vi "SV UFF58 Format ASCII Function (Complex Spectrum) (1 Ch).vi"(1 "ID lines (1-3)":T9, 2 "data precision (DBL:1)":T11=1 items=["single-precision", "double-precision"], 5 "real part":T10, 7 "imaginary part":T10, 9 "spectrum info":T1={"channel name"="", "description"="", "x-axis units"=0, "spectral info"={"spectrum type"=enum."Power [Magnitude^2]", "linear/dB"=enum."linear", "window"=0, "window size"=0, "FFT size"=0}, "engineering units"=0, "custom label"="", "dB reference [EU]"=0.0, "peak units"=enum."rms", "weighting filter"=0, "spectral density?"=FALSE, "unit label"="", "spectrum skewed?"=FALSE, "complimentary spectrum units"=enum."none"} {"x-axis units" items=["Time (s)"=0, "Frequency-CB (Hz)"=1, "Frequency-CPB (Hz)"=1248, "Frequency-Arbitrary (Hz)"=2357, "Quefrency (s)"=2, "Revolutions (rev)"=3, "Order"=4, "Speed (RPM)"=11, "Speed (rad/s)"=21, "Index"=65535]; "weighting filter" items=["Linear", "A-weighting", "B-weighting", "C-weighting", "ITU-R 468-4", "Dolby", "CCITT", "C-message", "Wb", "Wc", "Wd", "We", "Wf", "Wh", "Wj", "Wk", "Wm", "AES17 20 kHz lowpass", "AES17 40 kHz lowpass", "AES17 20 kHz highpass", "AES17 40 kHz highpass"]; "dB reference [EU]" format="%.2f"; "engineering units" items=["custom..."=0, "V"=1, "A"=21, "C"=30, "pC"=31, "s"=32, "-"=29, "Pa"=2, "N"=20, "g"=3, "m/s^2"=4, "m/s"=5, "m"=6, "mm/s"=12, "mm"=13, "micron/s"=14, "micron"=15, "in/s^2"=7, "in/s"=8, "in"=9, "mil/s"=10, "mil"=11, "rad/s^2"=16, "rad/s"=17, "rad"=18, "deg/s^2"=26, "deg/s"=27, "deg"=28, "RPM"=22, "cycle/s^2"=23, "Hz"=24, "cycle"=25, "strain"=19]; "spectral info"."window" items=["None "=0, "Hanning"=1, "Hamming"=2, "Blackman-Harris"=3, "Exact Blackman"=4, "Blackman"=5, "Flat Top"=6, "4 Term B-Harris "=7, "7 Term B-Harris"=8, "Low Sidelobe"=9, "Force - Exponential"=10, "Gaussian"=62]}, 11 "error in (no error)":errorcluster, 12 "DOF Identification":T8 {"reference direction" items=["-Z Rotation"=-6, "-Y Rotation"=-5, "-X Rotation"=-4, "-Z Translation"=-3, "-Y Translation"=-2, "-X Translation"=-1, "Scalar"=0, "+X Translation"=1, "+Y Translation"=2, "+Z Translation"=3, "+X Rotation"=4, "+Y Rotation"=5, "+Z Rotation"=6]; "response direction" items=["-Z Rotation"=-6, "-Y Rotation"=-5, "-X Rotation"=-4, "-Z Translation"=-3, "-Y Translation"=-2, "-X Translation"=-1, "Scalar"=0, "+X Translation"=1, "+Y Translation"=2, "+Z Translation"=3, "+X Rotation"=4, "+Y Rotation"=5, "+Z Rotation"=6]}) -> (6 "UFF58 ASCII function string":string, 15 "error out":errorcluster)   [LabVIEW 2017, in "SoundVib_UFF58.lvlib"]
doc: "Formats data to the UFF58 (universal file format) ASCII format. This VI also writes the fields in records 1, 2, and 3, <B>ID lines (1-3)</B> as well as all the records and fields associated with the specified instance and the attributes of input data. You can write a single time domain waveform, a single real frequency spectrum, or a complex frequency spectrum to a UFF58 formatted string. If a frequency spectrum is in decibels, this VI converts the spectrum to linear before writing the data to the formatted string. The default instance, SV UFF58 Format ASCII Function (Time Waveform), writes a single time domain waveform to the file specified by the <B>waveform</B> input. Wire data to the <B>waveform</B> input to determine the polymorphic instance to use or manually select the instance."
uses:
  <vilib>/addons/Sound and Vibration/svt_UFF58/SoundVib_UFF58.lvlib
  <vilib>/addons/Sound and Vibration/svt_UFF58/subVIs/sv_UFF58 Data Precision.ctl
  <vilib>/addons/Sound and Vibration/svt_UFF58/subVIs/sv_IDLines123.ctl
  <vilib>/addons/Sound and Vibration/svt_UFF58/subVIs/sv_UFF58 Response Direction.ctl
  <vilib>/addons/_NISVFA/_Shared subVIs/Controls/svc_Spectrum Info.ctl
  <vilib>/addons/_NISVFA/_Shared subVIs/Controls/svc_X-Axis Units.ctl
  <vilib>/addons/_NISVFA/_Shared subVIs/Controls/svc_Spectrum Type.ctl
  <vilib>/addons/_NISVFA/_Shared subVIs/Controls/svc_Engineering Units Text Ring.ctl
  <vilib>/addons/_NISVFA/_Shared subVIs/Controls/svc_Weighting Filter Text Ring.ctl
  <vilib>/addons/_NISVFA/_Shared subVIs/Controls/svc_Complimentary Spectrum Units.ctl
  <vilib>/addons/Sound and Vibration/svt_UFF58/subVIs/sv_UFF58 Check Data Valid (Freq - Complex) (1 Ch).vi
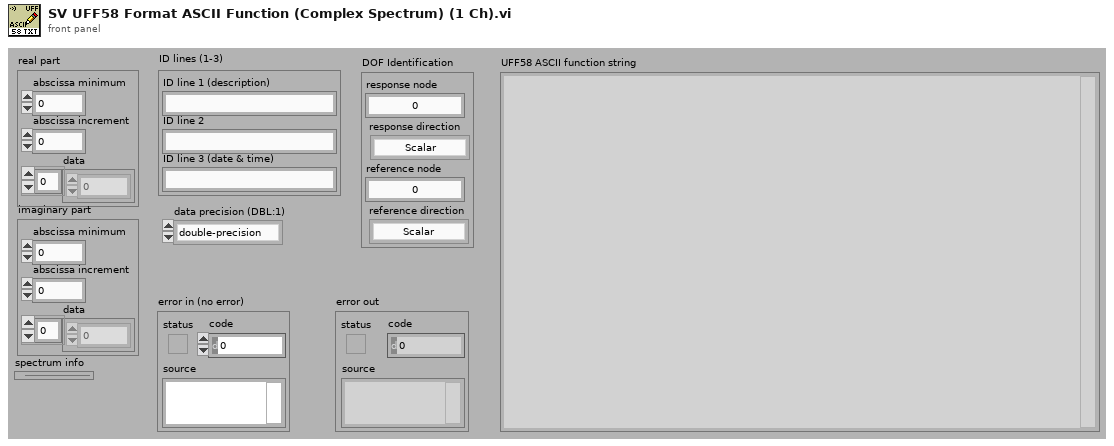
[diagram p1: front panel]
types:
  T1 = typedef "svc_Spectrum Info.ctl" = cluster{"channel name":string, "description":string, "x-axis units":T2, "spectral info":cluster{"spectrum type":T3, "linear/dB":enum16{"linear", "dB"}, "window":u16, "window size":i32, "FFT size":i32}, "engineering units":T4, "custom label":string, "dB reference [EU]":dbl, "peak units":enum16{"rms", "peak", "peak-peak"}, "weighting filter":T5, "spectral density?":bool, "unit label":string, "spectrum skewed?":bool, "complimentary spectrum units":T6}
  T2 = typedef "svc_X-Axis Units.ctl" = u16
  T3 = typedef "svc_Spectrum Type.ctl" = enum16{"FFT Spectrum [complex]", "Amplitude [Magnitude]", "Power [Magnitude^2]", "Cross Spectrum [complex]", "Frequency Response [Complex]"}
  T4 = typedef "svc_Engineering Units Text Ring.ctl" = u16
  T5 = typedef "svc_Weighting Filter Text Ring.ctl" = u16
  T6 = typedef "svc_Complimentary Spectrum Units.ctl" = enum16{"none", "radians", "degrees", "cycles", "imaginary"}
  T7 = typedef "SoundVib_UFF58.lvlib/sv_UFF58 Response Direction.ctl" = i32
  T8 = cluster{"response node":i32, "response direction":T7, "reference node":i32, "reference direction":T7}
  T9 = typedef "SoundVib_UFF58.lvlib/sv_IDLines123.ctl" = cluster{"ID line 1 (description)":string, "ID line 2":string, "ID line 3 (date & time)":string}
  T10 = cluster{"abscissa minimum":dbl, "abscissa increment":dbl, "data":dbl[]}
  T11 = typedef "SoundVib_UFF58.lvlib/sv_UFF58 Data Precision.ctl" = u32
  T12 = cluster{"record 1 - ID line 1 (description)":string, "record 2 - ID line 2":string, "record 3 - ID line 3 (date & time)":string, "record 4":string, "record 5":string}
  T13 = cluster{"ordinate data type":u16, "number of data values/pairs":i32, "abscissa spacing":enum16{"uneven", "even"}, "abscissa minimum":dbl, "abscissa increment":dbl, "z-axis value":dbl}
  T14 = typedef "SoundVib_UFF58.lvlib/sv_UFF58 DOF.ctl" = cluster{"function type":T15, "function ID number":i32, "version number":i32, "load case ID number":i32, "response entity name":string, "response node":i32, "response direction":T7, "reference entity name":string, "reference node":i32, "reference direction":T7}
  T15 = typedef "SoundVib_UFF58.lvlib/sv_FunctionType.ctl" = enum16{"general or unknown", "time response", "auto spectrum", "cross spectrum", "frequency response function", "transmissibility", "coherence", "auto correlation", "cross correlation", "power spectral density (PSD)", "energy spectral density (ESD)", "probability density function", "spectrum", "cumulative frequency distribution", "peaks valley", "stress/cycles", "strain/cycles", "orbit", "mode indicator function", "force pattern", "partial power", "partial coherence", "eigenvalue", "eigenvector", "shock response spectrum", "finite impulse response filter", "multiple coherence", "order function", "phase compensation"}
  T16 = typedef "SoundVib_UFF58.lvlib/sv_UFF58 Axis Characteristics.ctl" = cluster{"specific data type":T17, "length units exponent":i32, "force units exponent":i32, "temperature units exponent":i32, "axis label":string, "axis units label":string}
  T17 = typedef "SoundVib_UFF58.lvlib/sv_UFF58 Specific Datatype.ctl" = u16
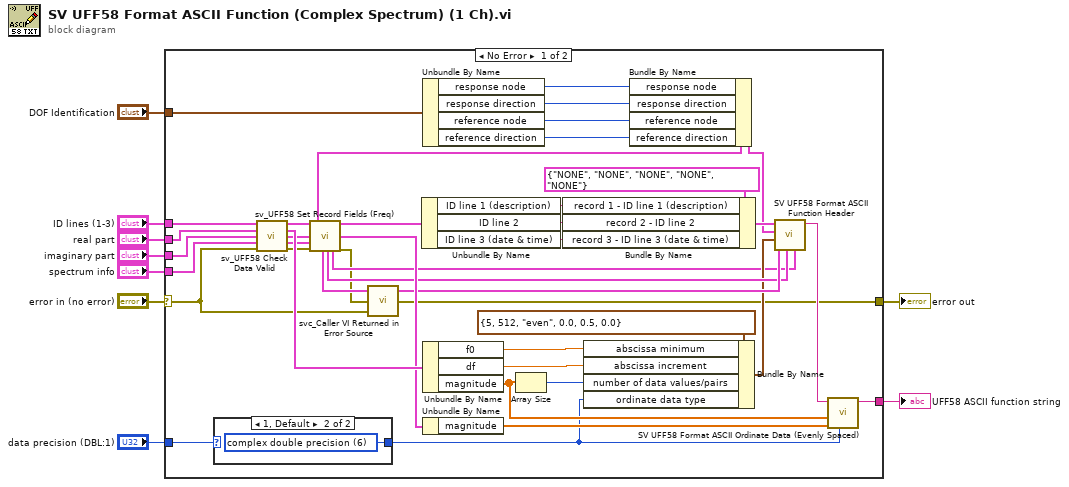
[diagram p0: block diagram]
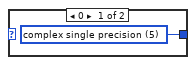
[diagram p2: hidden frame]
diagram:
  n1 = case shown="No Error" "error in (no error)" {
    selector: "error in (no error)" -> [w12 w50]
    tunnel: "data precision (DBL:1)" -> [w14 _]
    tunnel: [w44 _] -> w8
    tunnel: "real part" -> [w43 _]
    tunnel: "imaginary part" -> [w41 _]
    tunnel: "spectrum info" -> [w40 _]
    tunnel: "ID lines (1-3)" -> [w38 _]
    tunnel: "DOF Identification" -> [w36 _]
    tunnel: [w10 w50] -> w2
    frame No Error {
      n2 = case shown="1, Default" w14 {
        tunnel: [w48 w49] -> w13
        frame 0 {
          w48 = u16 5 items=["real single precision"=2, "real double precision"=4, "complex single precision"=5, "complex double precision"=6] ("ordinate data type")
        }
        frame 1, Default {
          w49 = u16 6 items=["real single precision"=2, "real double precision"=4, "complex single precision"=5, "complex double precision"=6] ("ordinate data type")
        }
      }
      n3 = call-poly <vilib>:"sv_UFF58 Check Data Valid.vi"("real part in"=w43, "imaginary part in"=w41, "spectrum info in"=w40, "error in (no error)"=w12) -> ("real part out"=w42:cluster{"f0":dbl, "df":dbl, "magnitude":dbl[]}, "imaginary part out"=w39:cluster{"f0":dbl, "df":dbl, "magnitude":dbl[]}, "spectrum info out"=w37:T1, "error out"=w24:errorcluster)  [unwired: 8 in]
      n4 = call <vilib>:"sv_UFF58 Set Record Fields (Freq).vi"("ID lines (1-3)"=w38, "spectrum info"=w37, "error in (no error)"=w24) -> ("DOF identification (record 6)"=w15:T14, "abscissa data characteristics (record 8)"=w33:T16, "ordinate numerator data characteristics (record 9)"=w32:T16, "ID lines (1-3) out"=w28:T9, "ordinate denominator data characteristics (record 10)"=w23:T16, "error out"=w11:errorcluster)  [unwired: 11 in]
      n5 = call <vilib>:"svc_Caller VI Returned in Error Source.vi"("warning input to caller"=w12, "error in (no error)"=w11) -> ("error out"=w10:errorcluster)  [unwired: 3 in]
      n6 = Unbundle By Name(w28) -> ("ID line 1 (description)"=w27:string, "ID line 2"=w26:string, "ID line 3 (date & time)"=w25:string)
      n7 = Unbundle By Name(w36) -> ("response node"=w35:i32, "response direction"=w34:T7, "reference node"=w18:i32, "reference direction"=w17:T7)
      n8 = Unbundle By Name(w42) -> ("f0"=w21:dbl, "df"=w20:dbl, "magnitude"=w22:dbl[])
      n9 = Unbundle By Name(w39) -> ("magnitude"=w46:dbl[])
      n10 = Array Size(array=w22) -> (size(s)=w19:i32)
      n11 = Bundle By Name(cluster=T12 {"record 1 - ID line 1 (description)"="NONE", "record 2 - ID line 2"="NONE", "record 3 - ID line 3 (date & time)"="NONE", "record 4"="NONE", "record 5"="NONE"} ("ID Lines 1-5"), "record 1 - ID line 1 (description)"=w27, "record 2 - ID line 2"=w26, "record 3 - ID line 3 (date & time)"=w25) -> (w29:T12)
      n12 = Bundle By Name(cluster=T13 {"ordinate data type"=5, "number of data values/pairs"=512, "abscissa spacing"=enum."even", "abscissa minimum"=0.0, "abscissa increment"=0.5, "z-axis value"=0.0} ("record 7 - data form"), "abscissa minimum"=w21, "abscissa increment"=w20, "number of data values/pairs"=w19, "ordinate data type"=w13) -> (w31:T13)
      n13 = Bundle By Name(cluster=w15, "response node"=w35, "response direction"=w34, "reference node"=w18, "reference direction"=w17) -> (w16:T14)
      n14 = call <vilib>:"SV UFF58 Format ASCII Function Header.vi"("record 10 - ordinate denominator data characteristics"=w23, "record 9 - ordinate data characteristics"=w32, "record 8 - abscissa data characteristics"=w33, "record 7 - data form"=w31, "record 6 - DOF identification"=w16, "records (1-5)"=w29) -> ("formatted UFF58 ASCII header"=w47:string)  [unwired: 5 in]
      n15 = call <vilib>:"SV UFF58 Format ASCII Ordinate Data (Evenly Spaced).vi"("ordinate data type"=w13, "ordinate values (Y Im)"=w46, "ordinate values (Y Re)"=w22, "formatted UFF58 ASCII header"=w47) -> ("UFF58 ASCII function string"=w44:string)  [unwired: 7 in]
    }
    frame Error {
    }
  }
  "UFF58 ASCII function string" <- w8
  "error out" <- w2
